vi "Absolute Accuracy Measurement.vi"(0 "VISA resource name":refnum<visa-resource-name>, 1 "Ae Accuracy (0.05)":dbl format="%.3f", 3 "Radcal":dbl format="%.2f", 5 "error in (no error)":errorcluster, 6 "Frequency (20)":dbl=20.0 min=20.0 max=1000000.0 format="%.2f") -> (11 "D Accuracy":dbl format="%^.2e", 13 "Q Accuracy":dbl format="%^.2e", 14 "VISA resource name out":refnum<visa-resource-name>, 15 "G Accuracy":dbl format="%^.2e", 16 "Rp Accuracy":dbl format="%^.2e", 17 "Rs Accuracy":dbl format="%^.2e", 18 "Deg Accuracy":dbl format="%^.2e", 19 "error out":errorcluster)   [LabVIEW 2015, in "Agilent 428X Series.lvlib"]
doc: "This VI calculate the absolute accuracy of the fllowing parameters:\nG,Q, Theta,D, Rs, and Rp.\nDa=De+Theta Cal\n\nDisclaimer: All accuracy calculation VI's are not part of the original \n driver. They are provided for supplementry purpose only.\n If user desires very high accuracy data, please do or \n check the calculation seperately."
uses:
  <instrlib>/Agilent 428X Series/Agilent 428X Series.lvlib
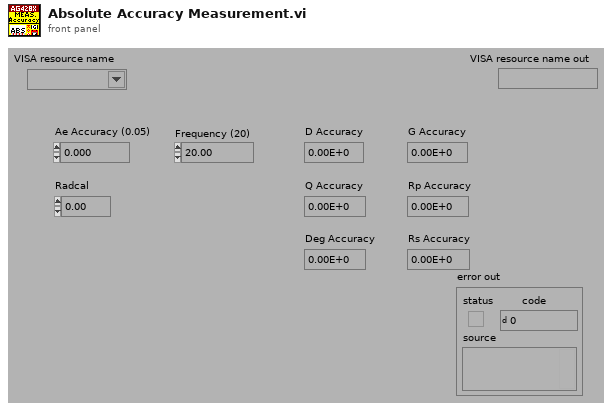
[diagram p1: front panel]
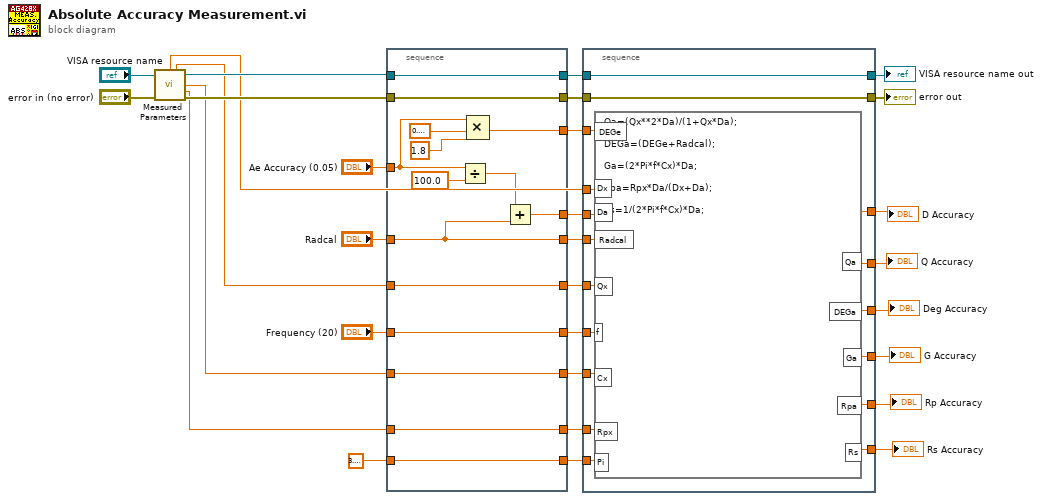
[diagram p0: block diagram]
diagram:
  n1 = call <instrlib>:"Measured Parameters.vi"("VISA resource name"="VISA resource name", "error in (no error)"="error in (no error)") -> ("Dx"=w11:dbl, "Qx"=w10:dbl, "VISA resource name out"=w13:refnum<visa-resource-name>, "Cx"=w7:dbl, "Rp"=w5:dbl, "error out"=w12:errorcluster)  [unwired: 7 in, 1 out]
  n2 = stacked-sequence {
    tunnel: [w45] -> w27
    tunnel: "Radcal" -> [w37]
    tunnel: "Ae Accuracy (0.05)" -> [w41]
    tunnel: w13 -> [w43]
    tunnel: w12 -> [w42]
    tunnel: [w43] -> w19
    tunnel: [w42] -> w17
    tunnel: [w38] -> w28
    tunnel: [w37] -> w25
    tunnel: w10 -> [w35]
    tunnel: [w35] -> w9
    tunnel: "Frequency (20)" -> [w34]
    tunnel: [w34] -> w1
    tunnel: w7 -> [w33]
    tunnel: [w33] -> w6
    tunnel: w5 -> [w32]
    tunnel: [w32] -> w4
    tunnel: 3.141592653589793 -> [w31]
    tunnel: [w31] -> w2
    frame #0 {
      n3 = Divide(x=w41, y=100.0) -> (x/y=w36:dbl)
      n4 = Compound Arithmetic op=MULTIPLY(w41, 0.3183098861837907, 1.8) -> (w38:dbl)
      n5 = Add(x=w36, y=w37) -> (x+y=w45:dbl)
    }
  }
  n6 = stacked-sequence {
    tunnel: w28 -> [w61]
    tunnel: w27 -> [w60]
    tunnel: [w60] -> w26
    tunnel: w9 -> [w59]
    tunnel: w25 -> [w58]
    tunnel: [w57] -> w24
    tunnel: [w56] -> w23
    tunnel: [w55] -> w22
    tunnel: [w54] -> w21
    tunnel: w11 -> [w53]
    tunnel: [w52] -> w20
    tunnel: w19 -> [w51]
    tunnel: [w51] -> w18
    tunnel: w17 -> [w50]
    tunnel: [w50] -> w16
    tunnel: w6 -> [w49]
    tunnel: w4 -> [w48]
    tunnel: w2 -> [w47]
    tunnel: w1 -> [w46]
    frame #0 {
      n7 = formula code="Qa=(Qx**2*Da)/(1+Qx*Da);\n\nDEGa=(DEGe+Radcal);\n\nGa=(2*Pi*f*Cx)*Da;\n\nRpa=Rpx*Da/(Dx+Da);\n\nRs=1/(2*Pi*f*Cx)*Da;"("DEGe"=w61, "Da"=w60, "Dx"=w53, "Qx"=w59, "f"=w46, "Cx"=w49, "Rpx"=w48, "Radcal"=w58, "Pi"=w47) -> ("Qa"=w57:dbl, "DEGa"=w56:dbl, "Ga"=w55:dbl, "Rpa"=w54:dbl, "Rs"=w52:dbl)
    }
  }
  "VISA resource name out" <- w18
  "error out" <- w16
  "D Accuracy" <- w26
  "Q Accuracy" <- w24
  "Deg Accuracy" <- w23
  "G Accuracy" <- w22
  "Rp Accuracy" <- w21
  "Rs Accuracy" <- w20
